vi "MTMount_getNextSample_CompressedAir.vi"(8 "error in (no error)":errorcluster, 11 "Compressed_Air_Ctl":T1) -> (0 "error out":errorcluster, 2 "function return":i32, 3 "Compressed_Air_Ctl out":T1)   [LabVIEW 2018, in "SALLV_MTMount.lvlib"]
doc: "int MTMount_shm_getNextSample_Compressed_AirLV(MTMount_Compressed_AirLV *Compressed_Air_Ctl );"
uses:
  SALLV_MTMount.lvlib
  DataTypes/Compressed_Air.ctl
  SALLV_MTMount.so
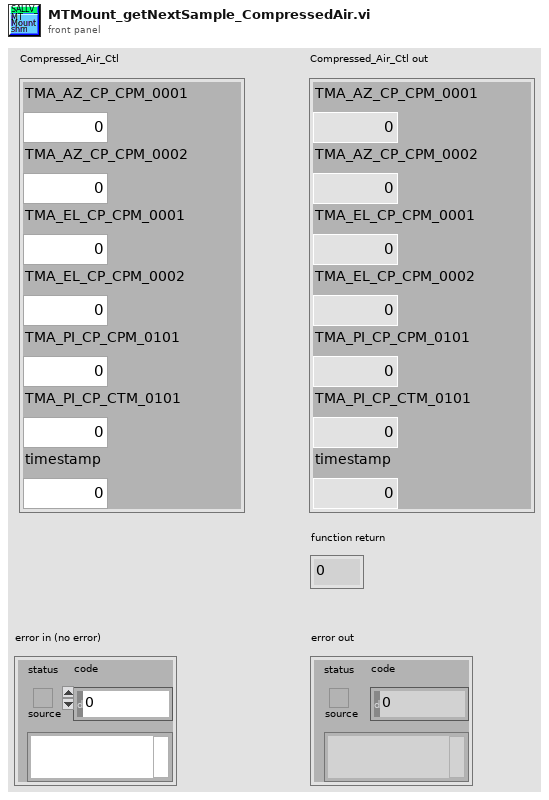
[diagram p1: front panel]
types:
  T1 = typedef "SALLV_MTMount.lvlib/Compressed_Air.ctl" = cluster{"TMA_AZ_CP_CPM_0001":dbl, "TMA_AZ_CP_CPM_0002":dbl, "TMA_EL_CP_CPM_0001":dbl, "TMA_EL_CP_CPM_0002":dbl, "TMA_PI_CP_CPM_0101":dbl, "TMA_PI_CP_CTM_0101":dbl, "timestamp":dbl}
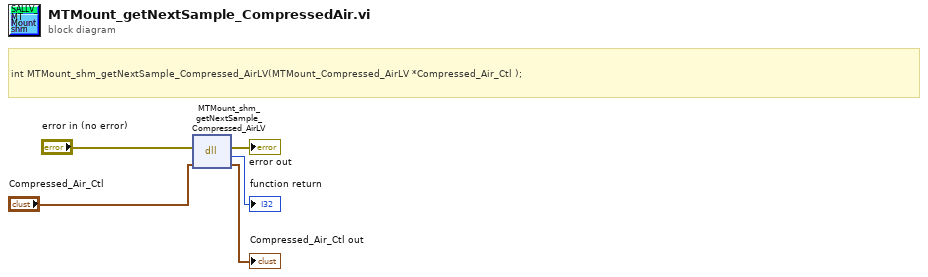
[diagram p0: block diagram]
diagram:
  # "int MTMount_shm_getNextSample_Compressed_AirLV(MTMount_Compressed_AirLV *Compressed_Air_Ctl );"
  n1 = dll-call lib="home/ttsai/Document/salApiMTMount/SALLV_MTMount/SALLV_MTMount.*" fn="MTMount_shm_getNextSample_Compressed_AirLV"(error in="error in (no error)", "Compressed_Air_Ctl"="Compressed_Air_Ctl") -> (error out=→"error out":errorcluster, →"function return":i32, "Compressed_Air_Ctl"=→"Compressed_Air_Ctl out":T1)  [unwired: 2 in, 1 out]
